vi "merge_PID.vi"   [LabVIEW 2017, in "NI_FunctionBlockMergeVIs.lvlib"]
doc: "PID algorithm for PID applications or high speed control applications that require an efficient algorithm. The PID algorithm features control output range limiting with integrator anti-windup and bumpless controller output for PID gain changes. This function block also features manual mode control with bumpless manual to automatic transitions, nonlinear integral action, two degree of freedom control, and error-squared control.\n\nYou can use this function block to operate on one input value at a time."
uses:
  <vilib>/functionblocks/NI_FunctionBlockMergeVIs.lvlib
  <vilib>/functionblocks/FB Core/FB Core.xnode
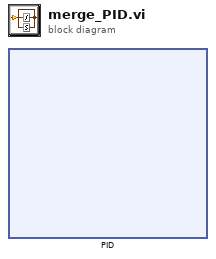
[diagram p0: block diagram]
diagram:
  n1 = xnode "PID"() -> ()  [unwired: 7 in, 2 out]
